vi "Step1to2.vi"   [LabVIEW 2019]
uses:
  Global Var.vi
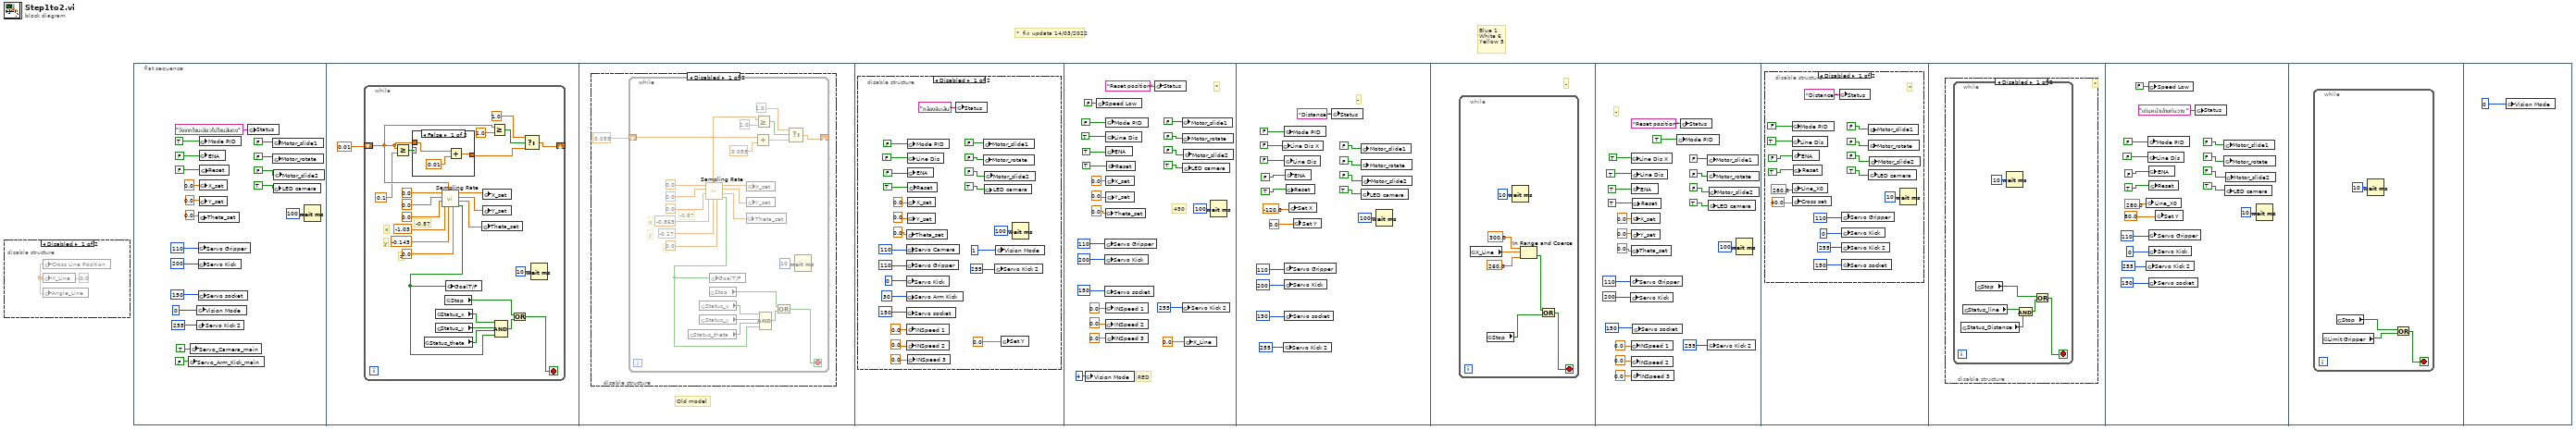
[diagram p0: block diagram]
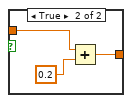
[diagram p3: hidden frame]
diagram:
  # "Blue 1\nWhite 6\nYellow 5"
  # "*  fix updata 14/03/2022"
  n1 = disable-structure shown="Disabled" {
    frame Disabled {
      w1 = 0.0 ("Cross Line Position")
      n2 = global write "Global Var.vi" "Cross Line Position"(w1) -> ()
      n3 = global write "Global Var.vi" "X_Line"(w1) -> ()
      n4 = global write "Global Var.vi" "Angle_Line"(w1) -> ()
    }
    frame Enabled {
    }
  }
  n5 = flat-sequence {
    frame #0 {
      n6 = global write "Global Var.vi" "Servo_Arm_Kick_main"(FALSE ("Mode PID")) -> ()
      n7 = global write "Global Var.vi" "Servo_Camera_main"(TRUE ("Mode PID")) -> ()
      n8 = global write "Global Var.vi" "Servo Kick 2"(u8 255 ("Servo Camera")) -> ()
      n9 = global write "Global Var.vi" "Vision Mode"(i16 0 ("Vision Mode")) -> ()
      n10 = global write "Global Var.vi" "Servo Gripper"(u8 110 ("Servo Camera")) -> ()
      n11 = global write "Global Var.vi" "Servo Kick"(u8 200 ("Servo Camera")) -> ()
      n12 = global write "Global Var.vi" "Servo socket"(u8 150 ("Servo Camera")) -> ()
      n13 = global write "Global Var.vi" "Theta_set"(0.0 ("Theta_set")) -> ()
      n14 = global write "Global Var.vi" "Mode PID"(TRUE ("Mode PID")) -> ()
      n15 = global write "Global Var.vi" "ENA"(FALSE ("ENA")) -> ()
      n16 = global write "Global Var.vi" "X_set"(0.0 ("X_set")) -> ()
      n17 = global write "Global Var.vi" "Y_set"(0.0 ("Y_set")) -> ()
      n18 = global write "Global Var.vi" "Reset"(FALSE ("ENA")) -> ()
      n19 = global write "Global Var.vi" "Status"("วิ่งจากโซนเขียวไปโซนสีแดง" ("Status")) -> ()
      n20 = global write "Global Var.vi" "Motor_slide1"(FALSE ("Mode PID")) -> ()
      n21 = global write "Global Var.vi" "Motor_rotate"(FALSE ("ENA")) -> ()
      n22 = global write "Global Var.vi" "LED camera"(TRUE ("LED camera")) -> ()
      n23 = global write "Global Var.vi" "Motor_slide2"(FALSE ("ENA")) -> ()
      n24 = Wait (ms)(milliseconds to wait=u32 100) -> ()  [unwired: 1 out]
    }
    frame #1 {
      n25 = while {
        shift-right: [w27] -> _
        shift-left: 0.01 -> [w23]
        stop <- w42 stop-if-true
        # "z"
        # "y"
        # "x"
        # "-0.87"
        n26 = Greater Or Equal?(x=w23, y=0.1) -> (x >= y?=w24:bool)
        n27 = case shown="False" w24 {
          tunnel: [w48 w51] -> w25
          tunnel: w23 -> [w47 w50]
          frame False {
            n28 = Add(x=w47, y=0.01) -> (x+y=w48:dbl)
          }
          frame True {
            n29 = Add(x=w50, y=0.2) -> (x+y=w51:dbl)
          }
        }
        n30 = global read "Global Var.vi" "Status_theta"() -> (w44:bool)
        n31 = global read "Global Var.vi" "Status_x"() -> (w45:bool)
        n32 = global read "Global Var.vi" "Status_y"() -> (w46:bool)
        n33 = call "Sampling Rate.vi"("input a1"=0.0, "input y1"=-0.145, "T(0-1)"=w23, "input x1"=-1.03, "input a0"=0.0, "input y0"=0.0, "input x0"=0.0) -> ("GoalT/F"=w30:bool, "a_output"=w37:dbl, "y_output"=w38:dbl, "x_output"=w39:dbl)  [unwired: 1 in]
        n34 = global read "Global Var.vi" "Stop"() -> (w40:bool)
        n35 = global write "Global Var.vi" "GoalT/F"(w30) -> ()
        n36 = global write "Global Var.vi" "Theta_set"(w37) -> ()
        n37 = global write "Global Var.vi" "X_set"(w39) -> ()
        n38 = global write "Global Var.vi" "Y_set"(w38) -> ()
        n39 = Greater Or Equal?(x=w23, y=1.0) -> (x >= y?=w29:bool)
        n40 = Compound Arithmetic op=AND(w45, w46, w44, w30) -> (w41:bool)
        n41 = Or(x=w40, y=w41) -> (x .or. y?=w42:bool)
        n42 = Select(t=1.0, s=w29, f=w25) -> (s? t:f=w27:dbl)
        n43 = Wait (ms)(milliseconds to wait=u32 10) -> ()  [unwired: 1 out]
      }
    }
    frame #2 {
      # "Old model"
      n44 = disable-structure shown="Disabled" {
        frame Disabled {
          n45 = while {
            shift-right: [w56] -> _
            shift-left: 0.055 -> [w54]
            stop <- w73 stop-if-true
            # "z"
            # "y"
            # "x"
            # "-0.87"
            n46 = global read "Global Var.vi" "Status_theta"() -> (w75:bool)
            n47 = global read "Global Var.vi" "Status_x"() -> (w76:bool)
            n48 = global read "Global Var.vi" "Status_y"() -> (w77:bool)
            n49 = call "Sampling Rate.vi"("input a1"=0.0, "input y1"=-0.17, "T(0-1)"=w54, "input x1"=-0.865, "input a0"=0.0, "input y0"=0.0, "input x0"=0.0) -> ("GoalT/F"=w61:bool, "a_output"=w68:dbl, "y_output"=w69:dbl, "x_output"=w70:dbl)  [unwired: 1 in]
            n50 = global read "Global Var.vi" "Stop"() -> (w71:bool)
            n51 = global write "Global Var.vi" "GoalT/F"(w61) -> ()
            n52 = global write "Global Var.vi" "Theta_set"(w68) -> ()
            n53 = global write "Global Var.vi" "X_set"(w70) -> ()
            n54 = global write "Global Var.vi" "Y_set"(w69) -> ()
            n55 = Add(x=w54, y=0.055) -> (x+y=w59:dbl)
            n56 = Greater Or Equal?(x=w54, y=1.0) -> (x >= y?=w58:bool)
            n57 = Compound Arithmetic op=AND(w76, w77, w75, w61) -> (w72:bool)
            n58 = Or(x=w71, y=w72) -> (x .or. y?=w73:bool)
            n59 = Select(t=1.0, s=w58, f=w59) -> (s? t:f=w56:dbl)
            n60 = Wait (ms)(milliseconds to wait=u32 10) -> ()  [unwired: 1 out]
          }
        }
        frame Enabled {
        }
      }
    }
    frame #3 {
      n61 = disable-structure shown="Disabled" {
        frame Disabled {
          n62 = global write "Global Var.vi" "Servo Camera"(u8 110 ("Servo Camera")) -> ()
          n63 = global write "Global Var.vi" "Servo Gripper"(u8 110 ("Servo Camera")) -> ()
          n64 = global write "Global Var.vi" "Servo Kick"(u8 0 ("Servo Camera")) -> ()
          n65 = global write "Global Var.vi" "Servo Arm Kick"(u8 30 ("Servo Camera")) -> ()
          n66 = global write "Global Var.vi" "Servo socket"(u8 150 ("Servo Camera")) -> ()
          n67 = global write "Global Var.vi" "Theta_set"(0.0 ("Theta_set")) -> ()
          n68 = global write "Global Var.vi" "INSpeed 1"(0.0 ("X_set")) -> ()
          n69 = global write "Global Var.vi" "INSpeed 2"(0.0 ("Y_set")) -> ()
          n70 = global write "Global Var.vi" "Mode PID"(FALSE ("Mode PID")) -> ()
          n71 = global write "Global Var.vi" "Line Dis"(FALSE ("Mode PID")) -> ()
          n72 = global write "Global Var.vi" "ENA"(FALSE ("ENA")) -> ()
          n73 = global write "Global Var.vi" "X_set"(0.0 ("X_set")) -> ()
          n74 = global write "Global Var.vi" "Y_set"(0.0 ("Y_set")) -> ()
          n75 = global write "Global Var.vi" "INSpeed 3"(0.0 ("Theta_set")) -> ()
          n76 = global write "Global Var.vi" "Reset"(TRUE ("ENA")) -> ()
          n77 = global write "Global Var.vi" "Status"("กล้องจับเส้น" ("Status")) -> ()
          n78 = global write "Global Var.vi" "Motor_slide1"(FALSE ("Mode PID")) -> ()
          n79 = global write "Global Var.vi" "Motor_rotate"(FALSE ("ENA")) -> ()
          n80 = global write "Global Var.vi" "LED camera"(TRUE ("LED camera")) -> ()
          n81 = global write "Global Var.vi" "Motor_slide2"(FALSE ("ENA")) -> ()
          n82 = global write "Global Var.vi" "Servo Kick 2"(u8 255 ("Servo Camera")) -> ()
          n83 = global write "Global Var.vi" "Vision Mode"(i16 1 ("Vision Mode")) -> ()
          n84 = global write "Global Var.vi" "Set Y"(0.0 ("Y_set")) -> ()
          n85 = Wait (ms)(milliseconds to wait=u32 100) -> ()  [unwired: 1 out]
        }
        frame Enabled {
        }
      }
    }
    frame #4 {
      # "RED"
      # "450"
      # "*"
      n86 = global write "Global Var.vi" "Vision Mode"(i16 4 ("Vision Mode")) -> ()
      n87 = global write "Global Var.vi" "Speed Low"(FALSE ("Speed Low")) -> ()
      n88 = global write "Global Var.vi" "Servo Gripper"(u8 110 ("Servo Camera")) -> ()
      n89 = global write "Global Var.vi" "Servo Kick"(u8 200 ("Servo Camera")) -> ()
      n90 = global write "Global Var.vi" "Servo socket"(u8 150 ("Servo Camera")) -> ()
      n91 = global write "Global Var.vi" "Theta_set"(0.0 ("Theta_set")) -> ()
      n92 = global write "Global Var.vi" "INSpeed 1"(0.0 ("X_set")) -> ()
      n93 = global write "Global Var.vi" "INSpeed 2"(0.0 ("Y_set")) -> ()
      n94 = global write "Global Var.vi" "Mode PID"(FALSE ("Mode PID")) -> ()
      n95 = global write "Global Var.vi" "Line Dis"(TRUE ("Mode PID")) -> ()
      n96 = global write "Global Var.vi" "ENA"(TRUE ("ENA")) -> ()
      n97 = global write "Global Var.vi" "X_set"(0.0 ("X_set")) -> ()
      n98 = global write "Global Var.vi" "Y_set"(0.0 ("Y_set")) -> ()
      n99 = global write "Global Var.vi" "INSpeed 3"(0.0 ("Theta_set")) -> ()
      n100 = global write "Global Var.vi" "Reset"(TRUE ("ENA")) -> ()
      n101 = global write "Global Var.vi" "Status"("Reset position" ("Status")) -> ()
      n102 = global write "Global Var.vi" "Motor_slide1"(FALSE ("Mode PID")) -> ()
      n103 = global write "Global Var.vi" "Motor_rotate"(FALSE ("ENA")) -> ()
      n104 = global write "Global Var.vi" "Servo Kick 2"(u8 255 ("Servo Camera")) -> ()
      n105 = global write "Global Var.vi" "LED camera"(TRUE ("LED camera")) -> ()
      n106 = global write "Global Var.vi" "Motor_slide2"(FALSE ("ENA")) -> ()
      n107 = global write "Global Var.vi" "X_Line"(0.0 ("X_set")) -> ()
      n108 = Wait (ms)(milliseconds to wait=u32 100) -> ()  [unwired: 1 out]
    }
    frame #5 {
      # "-"
      n109 = global write "Global Var.vi" "Line Dis X"(FALSE ("Mode PID")) -> ()
      n110 = global write "Global Var.vi" "Servo Kick 2"(u8 255 ("Servo Camera")) -> ()
      n111 = global write "Global Var.vi" "Mode PID"(FALSE ("Mode PID")) -> ()
      n112 = global write "Global Var.vi" "Servo Gripper"(u8 110 ("Servo Camera")) -> ()
      n113 = global write "Global Var.vi" "Servo Kick"(u8 200 ("Servo Camera")) -> ()
      n114 = global write "Global Var.vi" "Servo socket"(u8 150 ("Servo Camera")) -> ()
      n115 = global write "Global Var.vi" "Line Dis"(FALSE ("Mode PID")) -> ()
      n116 = global write "Global Var.vi" "ENA"(FALSE ("ENA")) -> ()
      n117 = global write "Global Var.vi" "Reset"(TRUE ("ENA")) -> ()
      n118 = global write "Global Var.vi" "Set X"(-120.0 ("Y_set")) -> ()
      n119 = global write "Global Var.vi" "Set Y"(0.0 ("Y_set")) -> ()
      n120 = global write "Global Var.vi" "Status"("Distance " ("Status")) -> ()
      n121 = global write "Global Var.vi" "Motor_slide1"(FALSE ("Mode PID")) -> ()
      n122 = global write "Global Var.vi" "Motor_rotate"(FALSE ("ENA")) -> ()
      n123 = global write "Global Var.vi" "LED camera"(TRUE ("LED camera")) -> ()
      n124 = global write "Global Var.vi" "Motor_slide2"(FALSE ("ENA")) -> ()
      n125 = Wait (ms)(milliseconds to wait=u32 100) -> ()  [unwired: 1 out]
    }
    frame #6 {
      # "-"
      n126 = while {
        stop <- w147 stop-if-true
        n127 = global read "Global Var.vi" "X_Line"() -> (w145:dbl)
        n128 = global read "Global Var.vi" "Stop"() -> (w146:bool)
        n129 = Wait (ms)(milliseconds to wait=u32 10) -> ()  [unwired: 1 out]
        n130 = In Range and Coerce(upper limit=300.0, x=w145, lower limit=260.0) -> (In Range?=w142:bool)  [unwired: 1 out]
        n131 = Or(x=w142, y=w146) -> (x .or. y?=w147:bool)
      }
    }
    frame #7 {
      # "-"
      n132 = global write "Global Var.vi" "Servo Gripper"(u8 110 ("Servo Camera")) -> ()
      n133 = global write "Global Var.vi" "Servo Kick"(u8 200 ("Servo Camera")) -> ()
      n134 = global write "Global Var.vi" "Line Dis X"(TRUE ("Mode PID")) -> ()
      n135 = global write "Global Var.vi" "Theta_set"(0.0 ("Theta_set")) -> ()
      n136 = global write "Global Var.vi" "INSpeed 1"(0.0 ("X_set")) -> ()
      n137 = global write "Global Var.vi" "INSpeed 2"(0.0 ("Y_set")) -> ()
      n138 = global write "Global Var.vi" "Line Dis"(TRUE ("Mode PID")) -> ()
      n139 = global write "Global Var.vi" "ENA"(TRUE ("ENA")) -> ()
      n140 = global write "Global Var.vi" "X_set"(0.0 ("X_set")) -> ()
      n141 = global write "Global Var.vi" "Y_set"(0.0 ("Y_set")) -> ()
      n142 = global write "Global Var.vi" "INSpeed 3"(0.0 ("Theta_set")) -> ()
      n143 = global write "Global Var.vi" "Reset"(TRUE ("ENA")) -> ()
      n144 = global write "Global Var.vi" "Servo socket"(u8 150 ("Servo Camera")) -> ()
      n145 = global write "Global Var.vi" "Mode PID"(TRUE ("Mode PID")) -> ()
      n146 = global write "Global Var.vi" "Status"("Reset position" ("Status")) -> ()
      n147 = global write "Global Var.vi" "Motor_slide1"(FALSE ("Mode PID")) -> ()
      n148 = global write "Global Var.vi" "Motor_rotate"(FALSE ("ENA")) -> ()
      n149 = global write "Global Var.vi" "Servo Kick 2"(u8 255 ("Servo Camera")) -> ()
      n150 = global write "Global Var.vi" "LED camera"(TRUE ("LED camera")) -> ()
      n151 = global write "Global Var.vi" "Motor_slide2"(FALSE ("ENA")) -> ()
      n152 = Wait (ms)(milliseconds to wait=u32 100) -> ()  [unwired: 1 out]
    }
    frame #8 {
      n153 = disable-structure shown="Disabled" {
        frame Disabled {
          # "*"
          n154 = global write "Global Var.vi" "Mode PID"(FALSE ("Mode PID")) -> ()
          n155 = global write "Global Var.vi" "Line Dis"(TRUE ("Mode PID")) -> ()
          n156 = global write "Global Var.vi" "ENA"(FALSE ("ENA")) -> ()
          n157 = global write "Global Var.vi" "Line_X0"(280.0 ("Y_set")) -> ()
          n158 = global write "Global Var.vi" "Cross set"(40.0 ("Y_set")) -> ()
          n159 = global write "Global Var.vi" "Reset"(TRUE ("ENA")) -> ()
          n160 = global write "Global Var.vi" "Status"("Distance " ("Status")) -> ()
          n161 = global write "Global Var.vi" "Servo Gripper"(u8 110 ("Servo Camera")) -> ()
          n162 = global write "Global Var.vi" "Servo Kick"(u8 0 ("Servo Camera")) -> ()
          n163 = global write "Global Var.vi" "Servo Kick 2"(u8 255 ("Servo Camera")) -> ()
          n164 = global write "Global Var.vi" "Servo socket"(u8 150 ("Servo Camera")) -> ()
          n165 = global write "Global Var.vi" "Motor_slide1"(FALSE ("Mode PID")) -> ()
          n166 = global write "Global Var.vi" "Motor_rotate"(FALSE ("ENA")) -> ()
          n167 = global write "Global Var.vi" "LED camera"(TRUE ("LED camera")) -> ()
          n168 = global write "Global Var.vi" "Motor_slide2"(FALSE ("ENA")) -> ()
          n169 = Wait (ms)(milliseconds to wait=u32 10) -> ()  [unwired: 1 out]
        }
        frame Enabled {
        }
      }
    }
    frame #9 {
      n170 = disable-structure shown="Disabled" {
        frame Disabled {
          # "*"
          n171 = while {
            stop <- w190 stop-if-true
            n172 = global read "Global Var.vi" "Status_Distance"() -> (w186:bool)
            n173 = global read "Global Var.vi" "Status_line"() -> (w187:bool)
            n174 = global read "Global Var.vi" "Stop"() -> (w189:bool)
            n175 = Wait (ms)(milliseconds to wait=u32 10) -> ()  [unwired: 1 out]
            n176 = And(x=w187, y=w186) -> (x .and. y?=w188:bool)
            n177 = Or(x=w189, y=w188) -> (x .or. y?=w190:bool)
          }
        }
        frame Enabled {
        }
      }
    }
    frame #10 {
      n178 = global write "Global Var.vi" "Line_X0"(280.0 ("Y_set")) -> ()
      n179 = global write "Global Var.vi" "Servo Kick 2"(u8 255 ("Servo Camera")) -> ()
      n180 = global write "Global Var.vi" "Mode PID"(FALSE ("Mode PID")) -> ()
      n181 = global write "Global Var.vi" "Line Dis"(FALSE ("Mode PID")) -> ()
      n182 = global write "Global Var.vi" "Speed Low"(FALSE ("Speed Low")) -> ()
      n183 = global write "Global Var.vi" "ENA"(FALSE ("ENA")) -> ()
      n184 = global write "Global Var.vi" "Servo Gripper"(u8 110 ("Servo Camera")) -> ()
      n185 = global write "Global Var.vi" "Servo Kick"(u8 0 ("Servo Camera")) -> ()
      n186 = global write "Global Var.vi" "Servo socket"(u8 150 ("Servo Camera")) -> ()
      n187 = global write "Global Var.vi" "Reset"(TRUE ("ENA")) -> ()
      n188 = global write "Global Var.vi" "Set Y"(80.0 ("Y_set")) -> ()
      n189 = global write "Global Var.vi" "Status"("เดินหน้าเข้าแท่นวาง " ("Status")) -> ()
      n190 = global write "Global Var.vi" "Motor_slide1"(FALSE ("Mode PID")) -> ()
      n191 = global write "Global Var.vi" "Motor_rotate"(FALSE ("ENA")) -> ()
      n192 = global write "Global Var.vi" "LED camera"(TRUE ("LED camera")) -> ()
      n193 = global write "Global Var.vi" "Motor_slide2"(FALSE ("ENA")) -> ()
      n194 = Wait (ms)(milliseconds to wait=u32 10) -> ()  [unwired: 1 out]
    }
    frame #11 {
      n195 = while {
        stop <- w211 stop-if-true
        n196 = global read "Global Var.vi" "Limit Gripper"() -> (w209:bool)
        n197 = global read "Global Var.vi" "Stop"() -> (w210:bool)
        n198 = Wait (ms)(milliseconds to wait=u32 10) -> ()  [unwired: 1 out]
        n199 = Or(x=w210, y=w209) -> (x .or. y?=w211:bool)
      }
    }
    frame #12 {
      n200 = global write "Global Var.vi" "Vision Mode"(i16 0 ("Vision Mode")) -> ()
    }
  }
